vi "Query the Page View for AUTO.vi"(8 "error in":errorcluster, 10 "Manual test number of Page View":u8 min=1 max=100, 11 "VISA resource name":refnum<visa-resource-name>) -> (0 "error out":errorcluster, 1 "Return the count of Page View String":u16, 2 "Return the Page View String":string, 3 "VISA resource name out":refnum<visa-resource-name>)   [LabVIEW 2011, in "GPT-9000.lvlib"]
uses:
  <instrlib>/GPT-9000/GPT-9000.lvlib
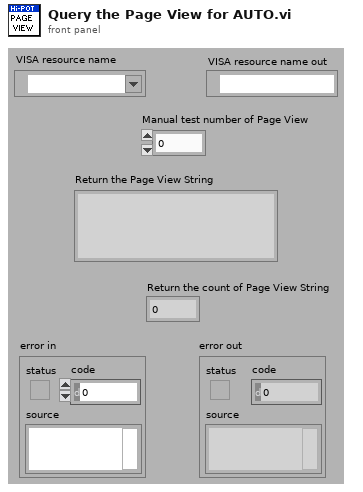
[diagram p1: front panel]
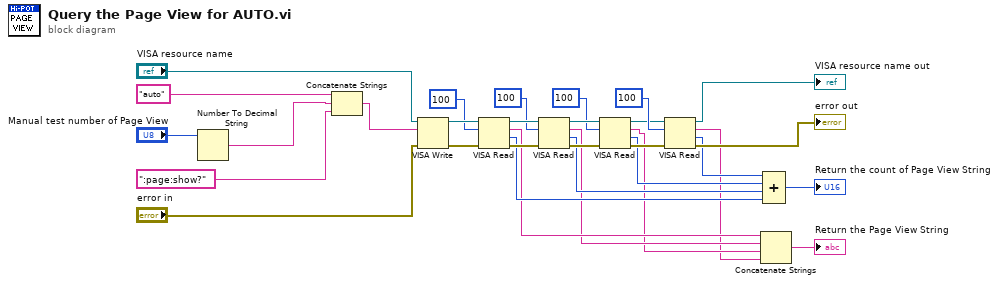
[diagram p0: block diagram]
diagram:
  n1 = Number To Decimal String(number="Manual test number of Page View") -> (decimal integer string=w29:string)  [unwired: 1 in]
  n2 = Concatenate Strings("auto", w29, ":page:show?") -> (w25:string)
  n3 = VISA Write(VISA resource name="VISA resource name", write buffer=w25, error in (no error)="error in") -> (VISA resource name out=w20:refnum<visa-resource-name>, error out=w21:errorcluster)  [unwired: 1 out]
  n4 = VISA Read(VISA resource name=w20, byte count=u32 100, error in (no error)=w21) -> (VISA resource name out=w18:refnum<visa-resource-name>, read buffer=w4:string, return count=w8:u32, error out=w19:errorcluster)
  n5 = VISA Read(VISA resource name=w18, byte count=u32 100, error in (no error)=w19) -> (VISA resource name out=w16:refnum<visa-resource-name>, read buffer=w3:string, return count=w7:u32, error out=w17:errorcluster)
  n6 = VISA Read(VISA resource name=w16, byte count=u32 100, error in (no error)=w17) -> (VISA resource name out=w12:refnum<visa-resource-name>, read buffer=w2:string, return count=w6:u32, error out=w11:errorcluster)
  n7 = VISA Read(VISA resource name=w12, byte count=u32 100, error in (no error)=w11) -> (VISA resource name out=→"VISA resource name out":refnum<visa-resource-name>, read buffer=w1:string, return count=w5:u32, error out=→"error out":errorcluster)
  n8 = Concatenate Strings(w4, w3, w2, w1) -> (→"Return the Page View String":string)
  n9 = Compound Arithmetic op=ADD(w5, w6, w7, w8) -> (→"Return the count of Page View String":u32)
